vi "Field within range V0.81.vi"(0 "ith step":u16, 1 "RampParameter":dbl[](array[numeric]) format="%.2f", 3 "Maximum Allowed Current":dbl format="%.2f", 4 "stopCycle":bool) -> (5 "Goto Field":dbl format="%.2f", 6 "Ramp Speed":dbl format="%.2f", 7 "Continue?":bool)   [LabVIEW 2025]
doc: "This Vi extract current field and set the scan continue boolean variable.\n\nThe field step can be either positive or negative.\n\nIf any of the absolute field value exceeds the maximum allowed limit, it will be replaced with the maximum field value itself\nAuthor: Scott Hannahs <sth@magnet.fsu.edu>\n\nThis software is licensed for use under the “MIT License\"\nCopyright (c) 2025 Scott Hannahs, sth@sth@magnet.sthnet.net\n\nPermission is hereby granted, free of charge, to any person obtaining a copy of this software and associated documentation files (the \"Software\"), to deal in the Software without restriction, including without limitation the rights to use, copy, modify, merge, publish, distribute, sublicense, and/or sell copies of the Software, and to permit persons to whom the Software is furnished to do so, subject to the following conditions: The above copyright notice and this permission notice shall be included in all copies or substantial portions of the Software.\n\nTHE SOFTWARE IS PROVIDED \"AS IS\", WITHOUT WARRANTY OF ANY KIND, EXPRESS OR IMPLIED, INCLUDING BUT NOT LIMITED TO THE WARRANTIES OF MERCHANTABILITY, FITNESS FOR A PARTICULAR PURPOSE AND NONINFRINGEMENT. IN NO EVENT SHALL THE AUTHORS OR COPYRIGHT HOLDERS BE LIABLE FOR ANY CLAIM, DAMAGES OR OTHER LIABILITY, WHETHER IN AN ACTION OF CONTRACT, TORT OR OTHERWISE, ARISING FROM, OUT OF OR IN CONNECTION WITH THE SOFTWARE OR THE USE OR OTHER DEALINGS IN THE SOFTWARE."
panel:
  out "Field Step":dbl format="%.2f"
  out "Final Field":dbl format="%.2f"
  out "Initial Field":dbl format="%.2f"
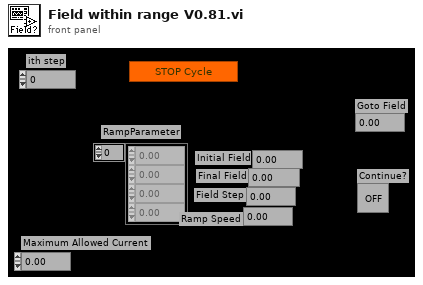
[diagram p1: front panel]
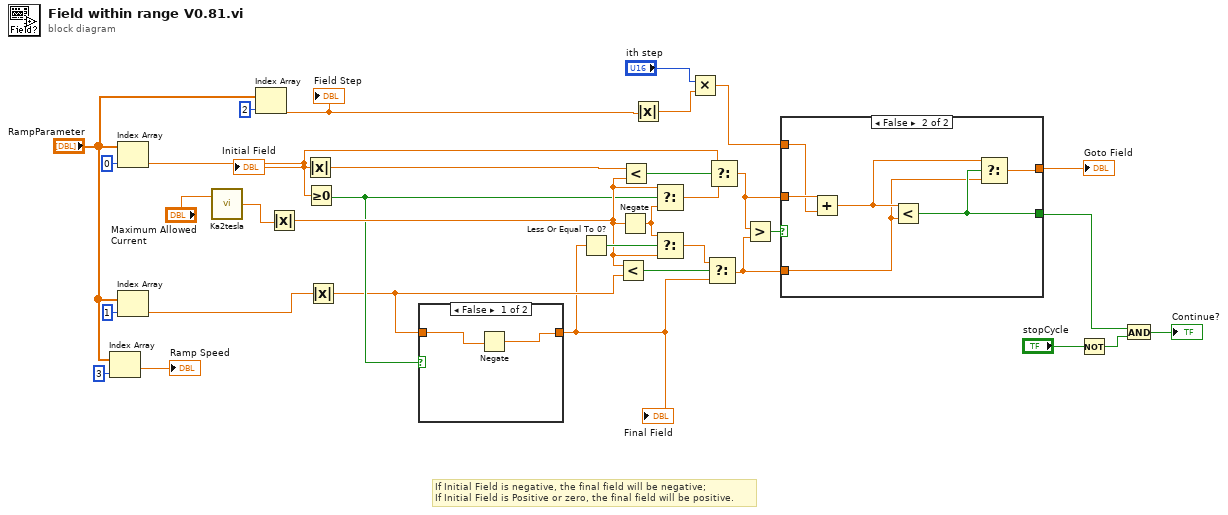
[diagram p0: block diagram]
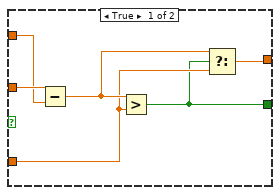
[diagram p3: hidden frame]
diagram:
  # "If Initial Field is negative, the final field will be negative;\nIf Initial Field is Positive or zero, the final field will be positive."
  n1 = Index Array(array="RampParameter", index=3) -> (element=→"Ramp Speed":dbl)
  n2 = Index Array(array="RampParameter", index=0) -> (element=w9:dbl)
  "Initial Field" <- w9
  n3 = Index Array(array="RampParameter", index=1) -> (element=w2:dbl)
  n4 = call "Ka2tesla.vi"("Magnet Current [kA]"="Maximum Allowed Current") -> ("Field"=w5:dbl)  [unwired: 1 in]
  n5 = Index Array(array="RampParameter", index=2) -> (element=w8:dbl)
  "Field Step" <- w8
  n6 = Absolute Value(x=w5) -> (abs(x)=w18:dbl)
  n7 = Absolute Value(x=w9) -> (abs(x)=w29:dbl)
  n8 = Greater Or Equal To 0?(x=w9) -> (x >= 0?=w4:bool)
  n9 = Absolute Value(x=w2) -> (abs(x)=w3:dbl)
  n10 = case shown="False" w4 {
    tunnel: w3 -> [w35 w36]
    tunnel: [w34 w36] -> w1
    frame False {
      n11 = Negate(x=w35) -> (-x=w34:dbl)
    }
    frame True {
    }
  }
  "Final Field" <- w1
  n12 = Less Or Equal To 0?(x=w1) -> (x <= 0?=w19:bool)
  n13 = Less?(x=w18, y=w3) -> (x < y?=w27:bool)
  n14 = Negate(x=w18) -> (-x=w17:dbl)
  n15 = Less?(x=w29, y=w18) -> (x < y?=w28:bool)
  n16 = Absolute Value(x=w8) -> (abs(x)=w25:dbl)
  n17 = Select(t=w18, s=w4, f=w17) -> (s? t:f=w20:dbl)
  n18 = Select(t=w17, s=w19, f=w18) -> (s? t:f=w16:dbl)
  n19 = Multiply(x="ith step", y=w25) -> (x*y=w22:dbl)
  n20 = Select(t=w16, s=w27, f=w1) -> (s? t:f=w23:dbl)
  n21 = Select(t=w9, s=w28, f=w20) -> (s? t:f=w24:dbl)
  n22 = Greater?(x=w24, y=w23) -> (0:w33:bool)
  n23 = case shown="False" w33 {
    tunnel: [w37 w45] -> w15
    tunnel: w24 -> [w42 w48]
    tunnel: w23 -> [w38 w44]
    tunnel: w22 -> [w41 w47]
    tunnel: [w40 w43] -> w21
    frame True {
      n24 = Subtract(x=w42, y=w41) -> (x-y=w39:dbl)
      n25 = Greater?(x=w39, y=w38) -> (0:w37:bool)
      n26 = Select(t=w39, s=w37, f=w38) -> (s? t:f=w40:dbl)
    }
    frame False {
      n27 = Add(x=w48, y=w47) -> (x+y=w46:dbl)
      n28 = Less?(x=w46, y=w44) -> (x < y?=w45:bool)
      n29 = Select(t=w46, s=w45, f=w44) -> (s? t:f=w43:dbl)
    }
  }
  "Goto Field" <- w21
  n30 = Not(x="stopCycle") -> (.not. x?=w32:bool)
  n31 = And(x=w15, y=w32) -> (x .and. y?=→"Continue?":bool)
